vi "remove_special_char_from_json.vi"(11 "JSON string":string) -> (3 "result string":string)   [LabVIEW 2015]
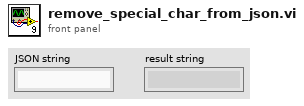
[diagram p1: front panel]
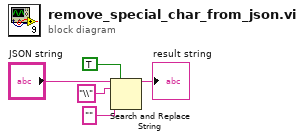
[diagram p0: block diagram]
diagram:
  n1 = Search and Replace String(replace all?=TRUE ("replace all? (F)"), input string="JSON string", search string="\\", replace string="" ("replace string (\"\")")) -> (result string=→"result string":string)  [unwired: 4 in, 3 out]
